vi "Read from FIFO.vi"(0 "FPGA VI Reference In":refnum<k20>, 1 "reset timestamp":bool, 2 "basic calc. interval (samples)":i32, 5 "number of channels":u8, 7 "poll time [ms]":i32=10, 11 "error in (no error)":errorcluster, 12 "half cycle (samples)":i32) -> (4 "AI data":sgl[][](array[numeric]) format="%#.21g", 6 "sample rate [Hz]":sgl=9600.0 format="%#.6g", 8 "RT controler time":timestamp, 14 "elements remaining":u32, 15 "error out":errorcluster)   [LabVIEW 2016]
uses:
  <vilib>/Analysis/baseanly.llb/Mean (DBL).vi
  <vilib>/Utility/error.llb/Error Cluster From Error Code.vi
  <vilib>/rvi/errors/niLvFpgaAdjustHostInterfaceError.vi
  <vilib>/rvi/interface/nirviMethod/nirviMethod.xnode
  <vilib>/FPGAPlugInAG/Dynamic/niLvFpga_ReadFifo_Dynamic.vi
  <vilib>/rvi/errors/niLvFpgaMergeErrorWithErrorCode.vi
  <vilib>/Analysis/NI_AALBase.lvlib
panel:
  in  "timeout (s)":dbl=5.0
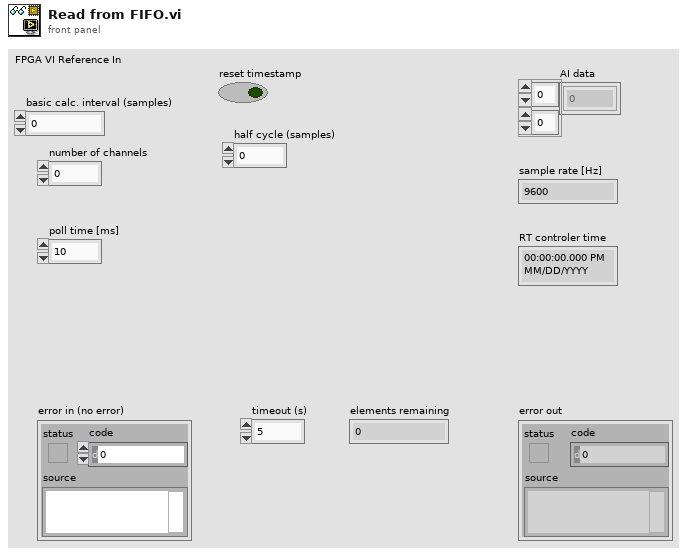
[diagram p1: front panel]
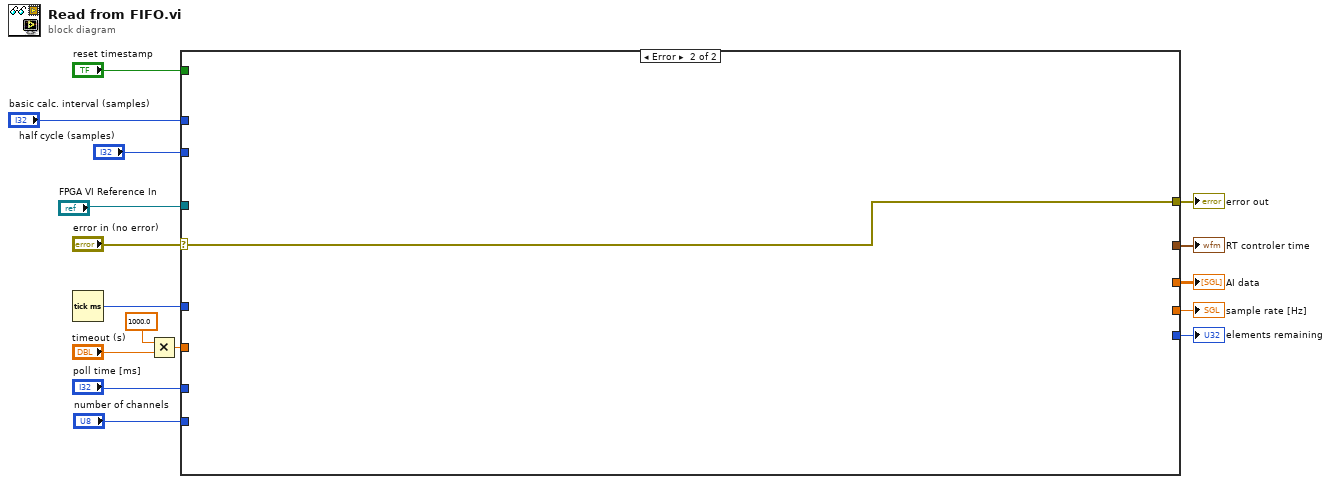
[diagram p0: block diagram]
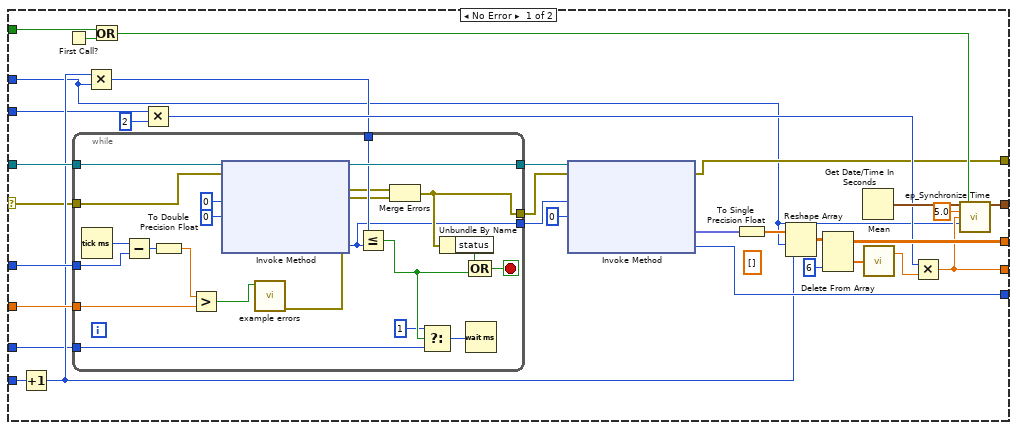
[diagram p2: hidden frame]
diagram:
  n1 = Tick Count (ms)() -> (millisecond timer value=w7:u32)
  n2 = Multiply(x=1000.0 ("y"), y="timeout (s)") -> (x*y=w6:dbl)
  n3 = case shown="Error" "error in (no error)" {
    selector: "error in (no error)" -> [w19 w71]
    tunnel: [w48 _] -> w16
    tunnel: [w47 _] -> w15
    tunnel: [w21 w71] -> w14
    tunnel: [w46 _] -> w13
    tunnel: [w45 _] -> w12
    tunnel: "FPGA VI Reference In" -> [w36 _]
    tunnel: "reset timestamp" -> [w27 _]
    tunnel: w7 -> [w35 _]
    tunnel: w6 -> [w44 _]
    tunnel: "number of channels" -> [w31 _]
    tunnel: "poll time [ms]" -> [w23 _]
    tunnel: "basic calc. interval (samples)" -> [w18 _]
    tunnel: "half cycle (samples)" -> [w17 _]
    frame No Error {
      (unwired) sgl[] [] ("single precision float")
      n4 = Increment(x=w31) -> (x+1=w25:u8)
      n5 = First Call?() -> (First Call?: T/F=w26:bool)
      n6 = Multiply(x=w25, y=w18) -> (x*y=w24:i32)
      n7 = while {
        tunnel: w35 -> [w68]
        tunnel: w44 -> [w65]
        tunnel: w19 -> [w63]
        tunnel: [w50] -> w32
        tunnel: [w59] -> w33
        tunnel: w36 -> [w60]
        tunnel: w24 -> [w58]
        tunnel: w23 -> [w54]
        tunnel: [w49] -> w20
        stop <- w61 stop-if-true
        n8 = Tick Count (ms)() -> (millisecond timer value=w70:u32)
        n9 = Subtract(x=w70, y=w68) -> (x-y=w69:u32)
        n10 = To Double Precision Float(number=w69) -> (double precision float=w66:dbl)
        n11 = Greater?(x=w66, y=w65) -> (0:w53:bool)
        n12 = xnode "Invoke Method"("FPGA VI Reference In"=w60, "error in"=w63, "Number of Elements"=u32 0, "Timeout (ms)"=0) -> ("FPGA VI Reference Out"=w59:refnum<k20>, "error out"=w52:errorcluster, "Elements Remaining"=w49:u32)  [unwired: 1 out]
        n13 = call <vilib>:"example errors.vi"("timeout?"=w53) -> ("error out"=w51:errorcluster)  [unwired: 10 in]
        n14 = Less Or Equal?(x=w58, y=w49) -> (x <= y?=w56:bool)
        n15 = Merge Errors(w52, w51) -> (w50:errorcluster)
        n16 = Select(t=1 ("index (row)"), s=w56, f=w54) -> (s? t:f=w57:i32)
        n17 = Unbundle By Name(w50) -> ("status"=w62:bool)
        n18 = Wait (ms)(milliseconds to wait=w57) -> ()  [unwired: 1 out]
        n19 = Compound Arithmetic op=OR(w62, w56) -> (w61:bool)
      }
      n20 = Or(x=w27, y=w26) -> (x .or. y?=w28:bool)
      n21 = Multiply(x=w17, y=2) -> (x*y=w29:i32)
      n22 = xnode "Invoke Method"("FPGA VI Reference In"=w33, "error in"=w32, "Number of Elements"=w20, "Timeout (ms)"=0) -> ("error out"=w21:errorcluster, "Data"=w43:fxp<+/-,26,5>[], "Elements Remaining"=w48:u32)  [unwired: 1 out]
      n23 = To Single Precision Float(number=w43) -> (single precision float=w41:sgl[])
      n24 = Reshape Array(w41, w18, w25) -> (w39:sgl[][])
      n25 = Delete From Array(array=w39, index (col)=6 ("index (row)")) -> (deleted portion=w42:sgl[], array with subset deleted=w47:sgl[][])  [unwired: 2 in]
      n26 = Get Date/Time In Seconds() -> (seconds since 1Jan1904=w40:timestamp)
      n27 = call-poly <vilib>:"Mean.vi"("X"=w42) -> ("mean"=w22:dbl)  [unwired: 1 out]
      n28 = Multiply(x=w29, y=w22) -> (x*y=w45:sgl)
      n29 = call <vilib>:"ep_Synchronize Time.vi"("RT controler time in"=w40, "reset"=w28, "maximum time difference (sec)"=5.0, "sampling rate (Hz)"=w45, "basic calc. interval (samples)"=w18) -> ("RT controler time out"=w46:timestamp)  [unwired: 10 in]
    }
    frame Error {
    }
  }
  "elements remaining" <- w16
  "RT controler time" <- w13
  "sample rate [Hz]" <- w12
  "AI data" <- w15
  "error out" <- w14
